vi "FormatTree&TableStyle.vi"(7 "Format Command":T1, 8 "Error In":errorcluster, 9 "Row Index":i32, 10 "Tbl Refnum":refnum<vi>, 11 "Tree Refnum":refnum<vi>) -> (0 "Error Out":errorcluster)   [LabVIEW 2012]
doc: "This VI implements the formatting of table data which includes highlighting, unhighlighting, and modifying visible rows (due to scrolling).\n\n<b>INPUTS</b>\n--------\n<b>Format Command </b> - Formatting action needs to be be taken\n<b>Table references array </b>- Array containing references of the tables of interest\n<b>Row </b>- Row number that needs to be fromatted"
uses:
  FormatTree&TableStyle_Commands.ctl
  <vilib>/Utility/miscctls.llb/LVRowAndColumnTypeDef.ctl
  <vilib>/Utility/miscctls.llb/LVRowAndColumnUnsignedTypeDef.ctl
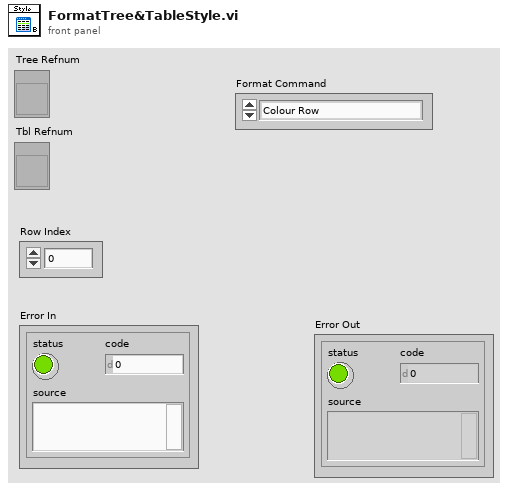
[diagram p1: front panel]
types:
  T1 = typedef "FormatTree&TableStyle_Commands.ctl" = enum16{"Colour Row", "Uncolour Row", "Bold Row", "Unbold Row", "Clear", "UpdateVisibleRows"}
  T2 = typedef "LVRowAndColumnTypeDef.ctl" = cluster{"Row":i32, "Column":i32}
  T3 = typedef "LVRowAndColumnUnsignedTypeDef.ctl" = cluster{"Row":u32, "Column":u32}
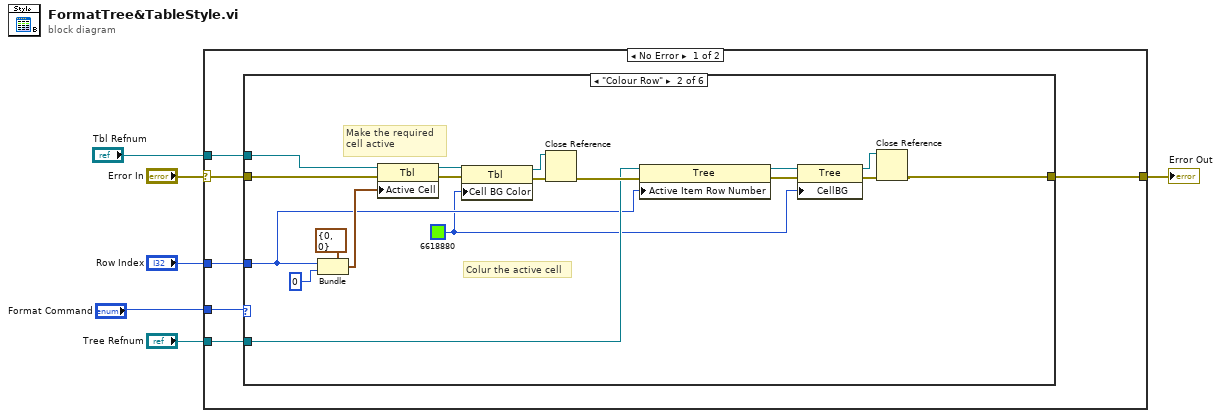
[diagram p0: block diagram]
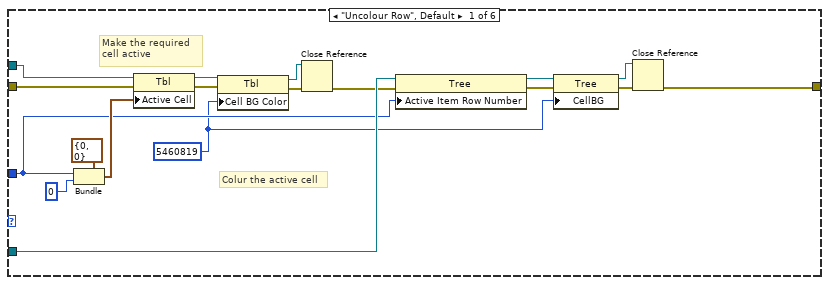
[diagram p2: hidden frame]
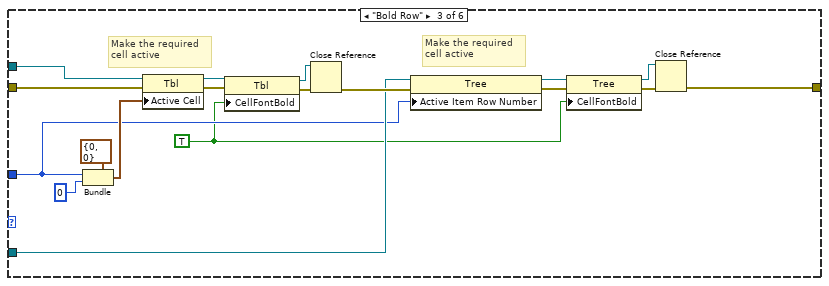
[diagram p3: hidden frame]
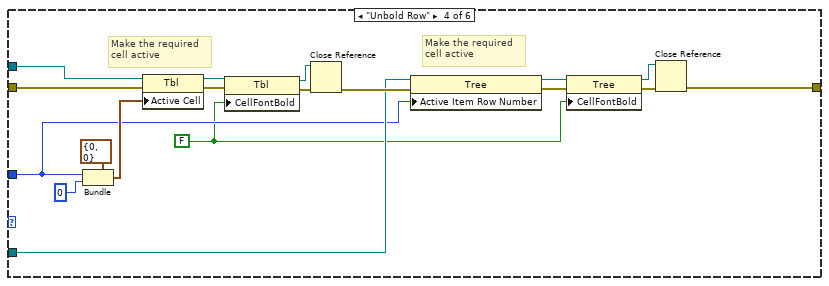
[diagram p4: hidden frame]
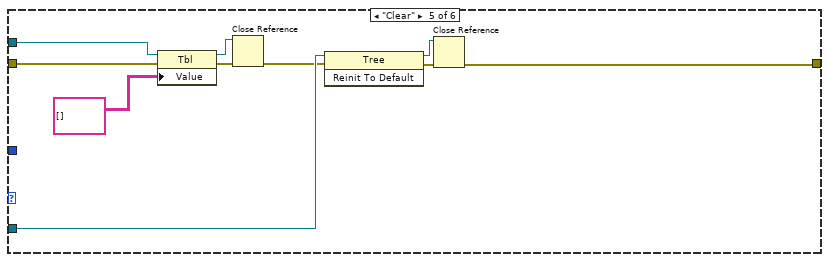
[diagram p5: hidden frame]
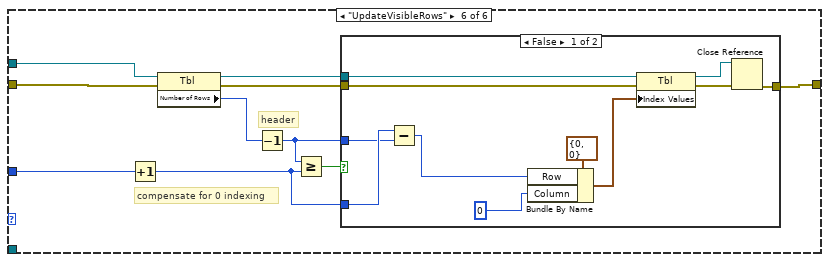
[diagram p6: hidden frame]
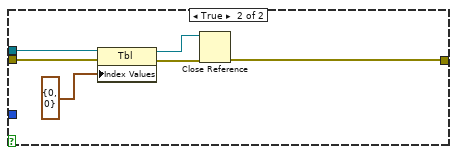
[diagram p7: hidden frame]
diagram:
  n1 = case shown="No Error" "Error In" {
    selector: "Error In" -> [w12 w122]
    tunnel: "Row Index" -> [w10 _]
    tunnel: [w9 w122] -> w4
    tunnel: "Tbl Refnum" -> [w11 _]
    tunnel: "Format Command" -> [w8 _]
    tunnel: "Tree Refnum" -> [w7 _]
    frame No Error {
      n2 = case shown="\"Colour Row\"" w8 {
        tunnel: w12 -> [w24 w36 w54 w72 w93 w103]
        tunnel: w11 -> [w23 w35 w53 w71 w94 w104]
        tunnel: w10 -> [w20 w33 w51 w69 _ w102]
        tunnel: [w14 w32 w50 w68 w85 w101] -> w9
        tunnel: w7 -> [w21 w34 w52 w70 w89 _]
        frame "Uncolour Row", Default {
          w13 = u32 5460819 ("Active Cell:Cell Background Color")
          # "Colur the active cell"
          # "Make the required cell active"
          n3 = Bundle(cluster=T2 {"Row"=0, "Column"=0} ("Active Cell:Active Cell"), "Row"=w20, "Column"=0) -> (w25:T2)
          n4 = property class="Tbl"(reference=w23, error in=w24, "Active Cell"=w25) -> (reference out=w30:refnum<vi>, error out=w29:errorcluster)
          n5 = property class="Tbl"(reference=w30, error in=w29, "Cell BG Color"=w13) -> (reference out=w27:refnum<vi>, error out=w28:errorcluster)
          n6 = Close Reference(reference=w27, error in (no error)=w28) -> (error out=w17:errorcluster)
          n7 = property class="Tree"(reference=w21, error in=w17, "Active Item Row Number"=w20) -> (reference out=w18:refnum<vi>, error out=w19:errorcluster)
          n8 = property class="Tree"(reference=w18, error in=w19, "CellBG"=w13) -> (reference out=w15:refnum<vi>, error out=w16:errorcluster)
          n9 = Close Reference(reference=w15, error in (no error)=w16) -> (error out=w14:errorcluster)
        }
        frame "Colour Row" {
          w31 = u32 6618880 ("Background colour")
          # "Colur the active cell"
          # "Make the required cell active"
          n10 = Bundle(cluster=T2 {"Row"=0, "Column"=0} ("Active Cell:Active Cell"), "Row"=w33, "Column"=0) -> (w43:T2)
          n11 = property class="Tbl"(reference=w35, error in=w36, "Active Cell"=w43) -> (reference out=w48:refnum<vi>, error out=w47:errorcluster)
          n12 = property class="Tbl"(reference=w48, error in=w47, "Cell BG Color"=w31) -> (reference out=w45:refnum<vi>, error out=w46:errorcluster)
          n13 = Close Reference(reference=w45, error in (no error)=w46) -> (error out=w39:errorcluster)
          n14 = property class="Tree"(reference=w34, error in=w39, "Active Item Row Number"=w33) -> (reference out=w40:refnum<vi>, error out=w41:errorcluster)
          n15 = property class="Tree"(reference=w40, error in=w41, "CellBG"=w31) -> (reference out=w37:refnum<vi>, error out=w38:errorcluster)
          n16 = Close Reference(reference=w37, error in (no error)=w38) -> (error out=w32:errorcluster)
        }
        frame "Bold Row" {
          w49 = TRUE ("Active Cell:Cell Font:Bold")
          # "Make the required cell active"
          # "Make the required cell active"
          n17 = Bundle(cluster=T2 {"Row"=0, "Column"=0} ("Active Cell:Active Cell"), "Row"=w51, "Column"=0) -> (w61:T2)
          n18 = property class="Tbl"(reference=w53, error in=w54, "Active Cell"=w61) -> (reference out=w66:refnum<vi>, error out=w65:errorcluster)
          n19 = property class="Tbl"(reference=w66, error in=w65, "CellFontBold"=w49) -> (reference out=w63:refnum<vi>, error out=w64:errorcluster)
          n20 = Close Reference(reference=w63, error in (no error)=w64) -> (error out=w57:errorcluster)
          n21 = property class="Tree"(reference=w52, error in=w57, "Active Item Row Number"=w51) -> (reference out=w58:refnum<vi>, error out=w59:errorcluster)
          n22 = property class="Tree"(reference=w58, error in=w59, "CellFontBold"=w49) -> (reference out=w55:refnum<vi>, error out=w56:errorcluster)
          n23 = Close Reference(reference=w55, error in (no error)=w56) -> (error out=w50:errorcluster)
        }
        frame "Unbold Row" {
          w67 = FALSE ("Active Cell:Cell Font:Bold")
          # "Make the required cell active"
          # "Make the required cell active"
          n24 = Bundle(cluster=T2 {"Row"=0, "Column"=0} ("Active Cell:Active Cell"), "Row"=w69, "Column"=0) -> (w79:T2)
          n25 = property class="Tbl"(reference=w71, error in=w72, "Active Cell"=w79) -> (reference out=w84:refnum<vi>, error out=w83:errorcluster)
          n26 = property class="Tbl"(reference=w84, error in=w83, "CellFontBold"=w67) -> (reference out=w81:refnum<vi>, error out=w82:errorcluster)
          n27 = Close Reference(reference=w81, error in (no error)=w82) -> (error out=w75:errorcluster)
          n28 = property class="Tree"(reference=w70, error in=w75, "Active Item Row Number"=w69) -> (reference out=w76:refnum<vi>, error out=w77:errorcluster)
          n29 = property class="Tree"(reference=w76, error in=w77, "CellFontBold"=w67) -> (reference out=w73:refnum<vi>, error out=w74:errorcluster)
          n30 = Close Reference(reference=w73, error in (no error)=w74) -> (error out=w68:errorcluster)
        }
        frame "Clear" {
          n31 = property class="Tbl"(reference=w94, error in=w93, "Value"=string[][] []) -> (reference out=w90:refnum<vi>, error out=w92:errorcluster)
          n32 = Close Reference(reference=w90, error in (no error)=w92) -> (error out=w88:errorcluster)
          n33 = invoke class="Tree" method="Reinit To Default"(reference=w89, error in=w88) -> (reference out=w86:refnum<vi>, error out=w87:errorcluster)  [unwired: 1 in, 1 out]
          n34 = Close Reference(reference=w86, error in (no error)=w87) -> (error out=w85:errorcluster)
        }
        frame "UpdateVisibleRows" {
          # "compensate for 0 indexing"
          # "header"
          n35 = Increment(x=w102) -> (x+1=w97:i32)
          n36 = property class="Tbl"(reference=w104, error in=w103) -> (reference out=w98:refnum<vi>, error out=w99:errorcluster, "Number of Rows"=w96:u32)
          n37 = Decrement(x=w96) -> (x-1=w95:u32)
          n38 = Greater Or Equal?(x=w95, y=w97) -> (x >= y?=w100:bool)
          n39 = case shown="False" w100 {
            tunnel: w99 -> [w114 w120]
            tunnel: w98 -> [w115 w121]
            tunnel: [w112 w117] -> w101
            tunnel: w95 -> [w106 _]
            tunnel: w97 -> [w107 _]
            frame False {
              n40 = Subtract(x=w107, y=w106) -> (x-y=w105:u32)
              n41 = Bundle By Name(cluster=T3 {"Row"=0, "Column"=0} ("Index Values"), "Row"=w105, "Column"=u32 0) -> (w108:T3)
              n42 = property class="Tbl"(reference=w115, error in=w114, "Index Values"=w108) -> (reference out=w110:refnum<vi>, error out=w111:errorcluster)
              n43 = Close Reference(reference=w110, error in (no error)=w111) -> (error out=w112:errorcluster)
            }
            frame True {
              n44 = property class="Tbl"(reference=w121, error in=w120, "Index Values"=T3 {"Row"=0, "Column"=0}) -> (reference out=w116:refnum<vi>, error out=w118:errorcluster)
              n45 = Close Reference(reference=w116, error in (no error)=w118) -> (error out=w117:errorcluster)
            }
          }
        }
      }
    }
    frame Error {
    }
  }
  "Error Out" <- w4
